vi "Query Spectrum Emission Offset FFT Width.vi"(0 "VISA resource name":refnum<visa-resource-name>, 11 "error in (no error)":errorcluster) -> (4 "VISA resource name out":refnum<visa-resource-name>, 6 "FFT Width":dbl[](array[numeric]), 15 "error out":errorcluster)   [LabVIEW 2020, in "Anritsu Signal Analyzer Series.lvlib"]
doc: "Queries the FFT width that is actually used for the sweep/FFT switch rule during offset measurement in the Spectrum Emission Mask measurement."
uses:
  Anritsu Signal Analyzer Series.lvlib
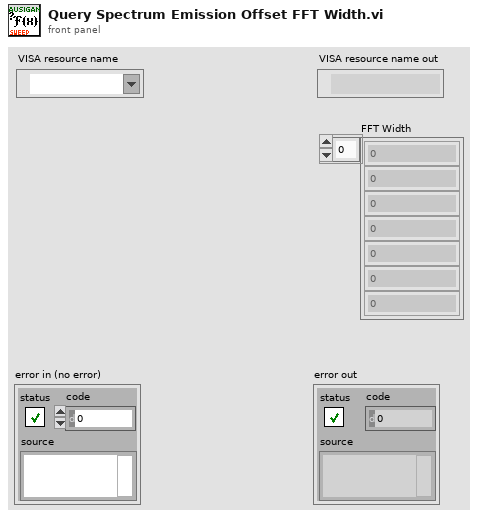
[diagram p1: front panel]
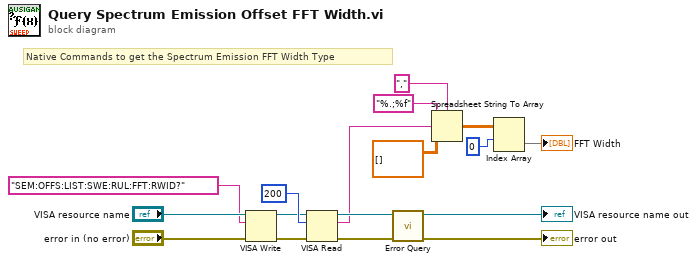
[diagram p0: block diagram]
diagram:
  # "Native Commands to get the Spectrum Emission FFT Width Type"
  n1 = VISA Write(VISA resource name="VISA resource name", write buffer="SEM:OFFS:LIST:SWE:RUL:FFT:RWID?" ("_Command"), error in (no error)="error in (no error)") -> (VISA resource name out=w11:refnum<visa-resource-name>, error out=w12:errorcluster)  [unwired: 1 out]
  n2 = VISA Read(VISA resource name=w11, byte count=u32 200 ("byte count (0)"), error in (no error)=w12) -> (VISA resource name out=w9:refnum<visa-resource-name>, read buffer=w7:string, error out=w10:errorcluster)  [unwired: 1 out]
  n3 = call "Error Query.vi"("error in (no error)"=w10, "VISA resource name"=w9) -> ("error out"=→"error out":errorcluster, "VISA resource name out"=→"VISA resource name out":refnum<visa-resource-name>)  [unwired: 6 in, 2 out]
  n4 = Spreadsheet String To Array(delimiter (Tab)=",", format string="%.;%f", spreadsheet string=w7, array type (2D Dbl)=dbl[][] []) -> (array=w3:dbl[][])
  n5 = Index Array(array=w3, index (row)=0) -> (element=→"FFT Width":dbl[])  [unwired: 1 in]
